vi "Sequence_var.vi"() -> ()   [LabVIEW 2019]
panel:
  in  "Sequence":dbl[](array[numeric])
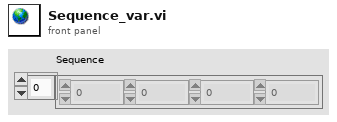
[diagram p1: front panel]
diagram:
